vi "FTW-Test-Reflection-ConPaneInterface.vi"() -> (0 "Test Result":errorcluster)   [LabVIEW 2015]
uses:
  src/reflection/FTW-Reflection-Types.ctl
  src/reflection/core/FTW-Reflection-ConPaneInterface-Function.ctl
  src/reflection/core/FTW-Reflection-ConPaneInterface-Terminal.ctl
  src/reflection/FTW-Reflection-Type.vi
  src/error/FTW-ERR-Assert-DeveloperError.vi
  src/error/FTW-ERR-StatusOK.vi
  src/reflection/FTW-Reflection-TypeDescriptorToDefaultData.vi
  src/error/FTW-ERR-NoErrorConstant.vi
  src/error/FTW-ERR-ThrowInfo.vi
  src/error/FTW-ERR-ThrowError.vi
  src/reflection/FTW-Reflection-Array.vi
  src/error/FTW-ERR-CallChain.vi
  src/string/FTW-STR-ReplaceWhitespace.vi
  src/string/FTW-STR-Array-Delimit.vi
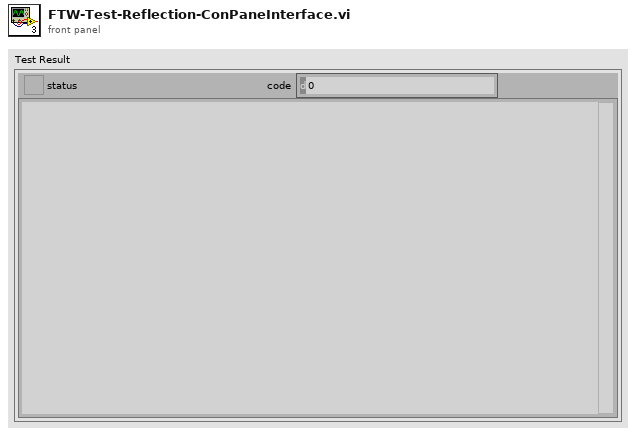
[diagram p1: front panel]
types:
  T1 = typedef "FTW-Reflection-ConPaneInterface-Terminal.ctl" = cluster{"Name":string, "LabVIEW Type":T2, "Datatype":variant, "Bounds":cluster{"Left":i32, "Top":i32, "Right":i32, "Bottom":i32}, "Input Stomp Index":i32, "Input":bool, "Wired":bool, "Dynamic Dispatch":bool, "Recommended":bool, "Required":bool, "Stomped":bool, "RSV20":bool, "RSV40":bool}
  T2 = typedef "FTW-Reflection-Types.ctl" = enum16{"Unknown", "Void", "Array", "Cluster", "LVObject", "Boolean", "I8", "I16", "I32", "I64", "U8", "U16", "U32", "U64", "SGL", "DBL", "EXT", "CSG", "CDB", "CXT", "FXP", "EnumU8", "EnumU16", "EnumU32", "EnumU64", "SGLwithUnit", "DBLwithUnit", "EXTwithUnit", "CSGwithUnit", "CDBwithUnit", "CXTwithUnit", "String", "Path", "Picture", "Tag", "LVVariant", "Timestamp", "WaveformI8", "WaveformI16", "WaveformI32", "WaveformI64", "WaveformU8", "WaveformU16", "WaveformU32", "WaveformU64", "WaveformSGL", "WaveformDBL", "WaveformEXT", "WaveformCSG", "WaveformCDB", "WaveformCXT", "WaveformDigital", "WaveformUnknownType", "DigitalData", "DynamicData", "ExternalData", "FileByteStream", "TDMStream", "dotNET", "ActiveX", "VIServerReference", "VIReference", "ApplicationInstance", "Menu", "ConnectionDataSocket", "ConnectionVISA", "ConnectionBluetooth", "ConnectionIrDA", "ConnectionTCP", "ConnectionUDP", "ConnectionHTTPClient", "ConnectionFTP", "Occurrence", "Notifier", "Queue", "Rendezvous", "Semaphore", "RTFIFO", "EventPublisher", "EventRegistration", "EventCallback", "DataValueReference", "GenericClass", "GenericClassTag", "GenericClassDeepCopy", "GenericClassFlattened", "GenericClassTagFlattened", "GenericReferenceType", "WindowsRegistry", "OverloadedDatalogRef", "ReferenceUnknownType", "ByteArray", "ConPaneInterface", "FTWObject"}
  T3 = typedef "FTW-Reflection-ConPaneInterface-Function.ctl" = cluster{"ConPane Code":i32, "ConPane Rotated":bool, "ConPane Flipped Horizontally":bool, "Asynchronous":bool, "Not a Pure Function (has side effects), or not SubRoutine":bool, "Subroutine Priority":bool, "Reserved 1":bool, "Reserved 2":bool, "Reserved 3":bool, "Reserved 4":bool, "Reserved 5":bool}
  T4 = cluster{i32, "ConPane Code":i32, "ConPane Rotated":bool, "ConPane Flipped Horizontally":bool}[]
  T5 = cluster{i32, "ConPane Code":i32, "ConPane Rotated":bool, "ConPane Flipped Horizontally":bool}
  T6 = cluster{"Name":string, "Wired":bool, "Required":bool, "Recommended":bool, "LabVIEW Type":T2}[]
  T7 = cluster{"Name":string, "Wired":bool, "Required":bool, "Recommended":bool, "LabVIEW Type":T2}
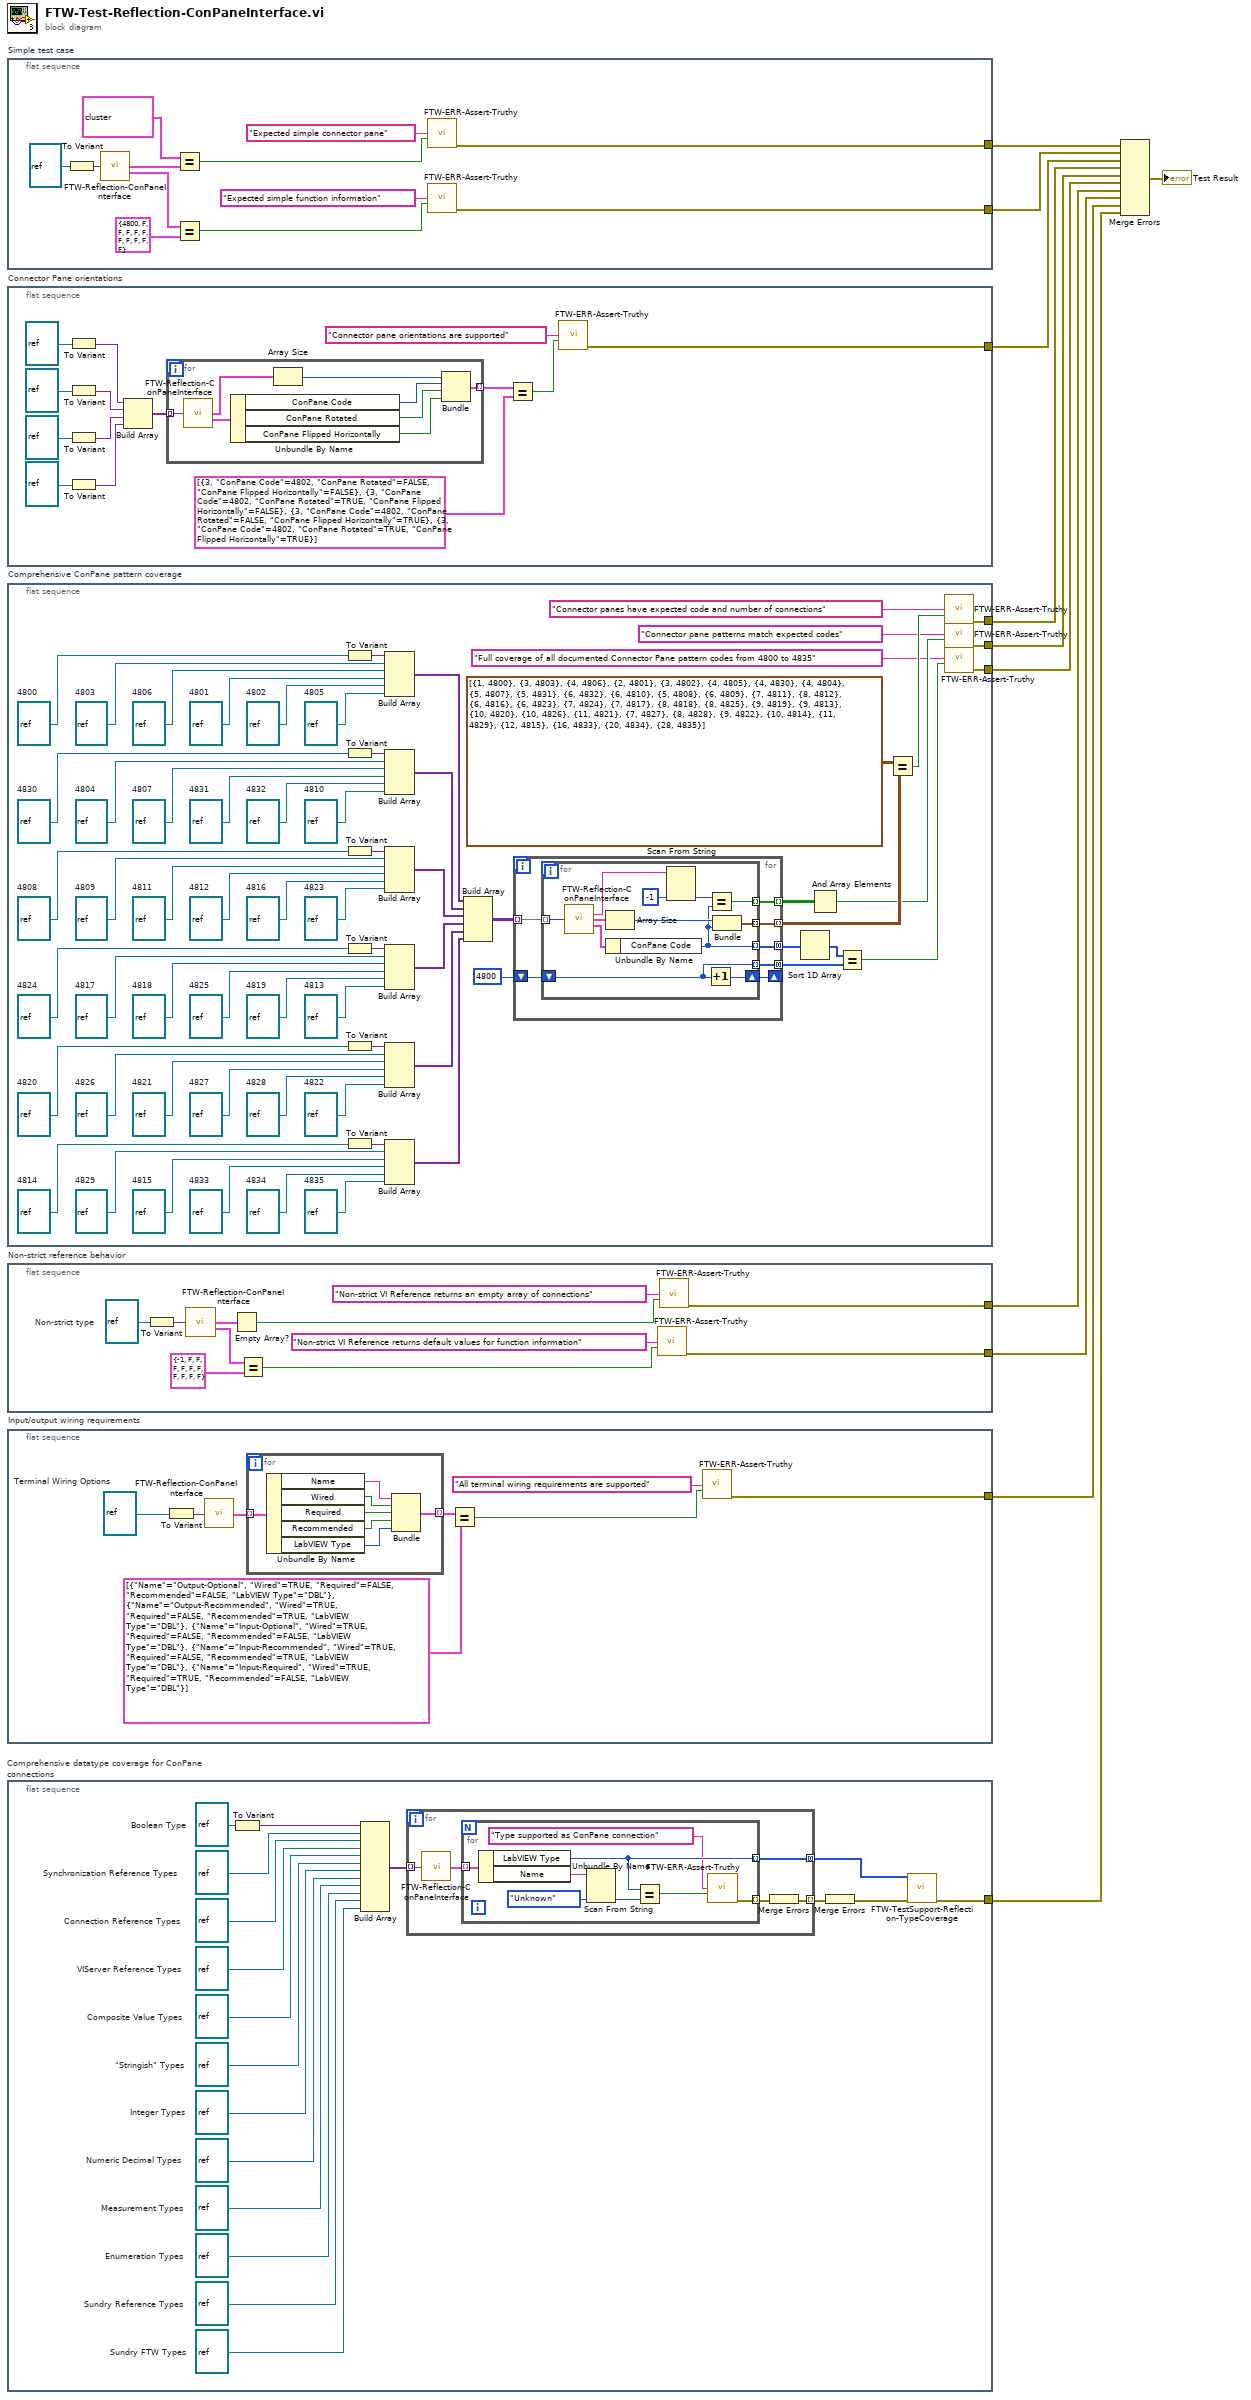
[diagram p0: block diagram]
diagram:
  n1 = flat-sequence "Simple test case" {
    tunnel: [w15] -> w11
    tunnel: [w12] -> w10
    frame #0 {
      n2 = To Variant(anything=refnum<vi> refnum) -> (Variant=w18:variant)
      n3 = call "FTW-Reflection-ConPaneInterface.vi"("VI Connector Pane (or VI Reference)"=w18) -> ("Terminals"=w23:T1[], "Function Information"=w21:T3)  [unwired: 12 in, 1 out]
      n4 = Equal?(x=T1[] [{"Name"="", "LabVIEW Type"=enum."Unknown", "Datatype"=variant, "Bounds"={"Left"=0, "Top"=0, "Right"=32, "Bottom"=32}, "Input Stomp Index"=-1, "Input"=FALSE, "Wired"=FALSE, "Dynamic Dispatch"=FALSE, "Recommended"=FALSE, "Required"=FALSE, "Stomped"=FALSE, "RSV20"=FALSE, "RSV40"=FALSE}] ("Terminals"), y=w23) -> (x = y?=w17:bool)
      n5 = Equal?(x=w21, y=T3 {"ConPane Code"=4800, "ConPane Rotated"=FALSE, "ConPane Flipped Horizontally"=FALSE, "Asynchronous"=FALSE, "Not a Pure Function (has side effects), or not SubRoutine"=FALSE, "Subroutine Priority"=FALSE, "Reserved 1"=FALSE, "Reserved 2"=FALSE, "Reserved 3"=FALSE, "Reserved 4"=FALSE, "Reserved 5"=FALSE} ("Function Information")) -> (x = y?=w13:bool)
      n6 = call "FTW-ERR-Assert-Truthy.vi"("Assertion"="Expected simple connector pane", "Assertion holds true?"=w17) -> ("error out"=w15:errorcluster)  [unwired: 13 in]
      n7 = call "FTW-ERR-Assert-Truthy.vi"("Assertion"="Expected simple function information", "Assertion holds true?"=w13) -> ("error out"=w12:errorcluster)  [unwired: 13 in]
    }
  }
  n8 = flat-sequence "Connector Pane orientations" {
    tunnel: [w24] -> w9
    frame #0 {
      n9 = To Variant(anything=refnum<vi> refnum) -> (Variant=w35:variant)
      n10 = To Variant(anything=refnum<vi> refnum) -> (Variant=w31:variant)
      n11 = To Variant(anything=refnum<vi> refnum) -> (Variant=w30:variant)
      n12 = To Variant(anything=refnum<vi> refnum) -> (Variant=w29:variant)
      n13 = Build Array(w35, w31, w30, w29) -> (w36:variant[])
      n14 = for {
        tunnel: [w41] -> w28 mode=indexing
        tunnel: w36 -> [w40] mode=indexing
        n15 = call "FTW-Reflection-ConPaneInterface.vi"("VI Connector Pane (or VI Reference)"=w40) -> ("Terminals"=w38:T1[], "Function Information"=w39:T3)  [unwired: 12 in, 1 out]
        n16 = Unbundle By Name(w39) -> ("ConPane Code"=w44:i32, "ConPane Rotated"=w43:bool, "ConPane Flipped Horizontally"=w42:bool)
        n17 = Array Size(array=w38) -> (size(s)=w45:i32)
        n18 = Bundle(w45, "ConPane Code"=w44, "ConPane Rotated"=w43, "ConPane Flipped Horizontally"=w42) -> (w41:T5)  [unwired: 1 in]
      }
      n19 = Equal?(x=w28, y=T4 [{3, "ConPane Code"=4802, "ConPane Rotated"=FALSE, "ConPane Flipped Horizontally"=FALSE}, {3, "ConPane Code"=4802, "ConPane Rotated"=TRUE, "ConPane Flipped Horizontally"=FALSE}, {3, "ConPane Code"=4802, "ConPane Rotated"=FALSE, "ConPane Flipped Horizontally"=TRUE}, {3, "ConPane Code"=4802, "ConPane Rotated"=TRUE, "ConPane Flipped Horizontally"=TRUE}] ("Array")) -> (x = y?=w25:bool)
      n20 = call "FTW-ERR-Assert-Truthy.vi"("Assertion"="Connector pane orientations are supported", "Assertion holds true?"=w25) -> ("error out"=w24:errorcluster)  [unwired: 13 in]
    }
  }
  n21 = flat-sequence "Comprehensive ConPane pattern coverage" {
    tunnel: [w48] -> w8
    tunnel: [w47] -> w7
    tunnel: [w46] -> w6
    frame #0 {
      w81 = refnum<vi> refnum  # 4835
      w86 = refnum<vi> refnum  # 4822
      w82 = refnum<vi> refnum  # 4834
      w87 = refnum<vi> refnum  # 4828
      w83 = refnum<vi> refnum  # 4833
      w88 = refnum<vi> refnum  # 4827
      w84 = refnum<vi> refnum  # 4815
      w89 = refnum<vi> refnum  # 4821
      w85 = refnum<vi> refnum  # 4829
      w90 = refnum<vi> refnum  # 4826
      w74 = refnum<vi> refnum  # 4814
      w73 = refnum<vi> refnum  # 4820
      w91 = refnum<vi> refnum  # 4813
      w96 = refnum<vi> refnum  # 4823
      w92 = refnum<vi> refnum  # 4819
      w97 = refnum<vi> refnum  # 4816
      w93 = refnum<vi> refnum  # 4825
      w98 = refnum<vi> refnum  # 4812
      w94 = refnum<vi> refnum  # 4818
      w99 = refnum<vi> refnum  # 4811
      w95 = refnum<vi> refnum  # 4817
      w100 = refnum<vi> refnum  # 4809
      w72 = refnum<vi> refnum  # 4824
      w71 = refnum<vi> refnum  # 4808
      w101 = refnum<vi> refnum  # 4810
      w106 = refnum<vi> refnum  # 4805
      w102 = refnum<vi> refnum  # 4832
      w107 = refnum<vi> refnum  # 4802
      w103 = refnum<vi> refnum  # 4831
      w108 = refnum<vi> refnum  # 4801
      w104 = refnum<vi> refnum  # 4807
      w109 = refnum<vi> refnum  # 4806
      w105 = refnum<vi> refnum  # 4804
      w110 = refnum<vi> refnum  # 4803
      w70 = refnum<vi> refnum  # 4830
      w62 = refnum<vi> refnum  # 4800
      n22 = To Variant(anything=w62) -> (Variant=w63:variant)
      n23 = To Variant(anything=w70) -> (Variant=w69:variant)
      n24 = To Variant(anything=w71) -> (Variant=w68:variant)
      n25 = To Variant(anything=w72) -> (Variant=w67:variant)
      n26 = To Variant(anything=w73) -> (Variant=w66:variant)
      n27 = To Variant(anything=w74) -> (Variant=w65:variant)
      n28 = Build Array(w63, w110, w109, w108, w107, w106) -> (w80:variant[])
      n29 = Build Array(w69, w105, w104, w103, w102, w101) -> (w79:variant[])
      n30 = Build Array(w68, w100, w99, w98, w97, w96) -> (w78:variant[])
      n31 = Build Array(w67, w95, w94, w93, w92, w91) -> (w77:variant[])
      n32 = Build Array(w66, w90, w89, w88, w87, w86) -> (w76:variant[])
      n33 = Build Array(w65, w85, w84, w83, w82, w81) -> (w75:variant[])
      n34 = Build Array(w80, w79, w78, w77, w76, w75) -> (w64:variant[][])
      n35 = for {
        tunnel: w64 -> [w117] mode=indexing
        tunnel: [w116] -> w56 mode=indexing
        tunnel: [w115] -> w61 mode=concatenating
        shift-right: [w113] -> _
        shift-left: 4800 ("ConPane Code") -> [w114]
        tunnel: [w112] -> w58 mode=concatenating
        tunnel: [w111] -> w55 mode=indexing
        n36 = for {
          tunnel: w117 -> [w129] mode=indexing
          tunnel: [w125] -> w116 mode=indexing
          tunnel: [w119] -> w115 mode=indexing
          shift-right: [w124] -> w113
          shift-left: w114 -> [w123]
          tunnel: [w123] -> w112 mode=indexing
          tunnel: [w118] -> w111 mode=indexing
          n37 = call "FTW-Reflection-ConPaneInterface.vi"("VI Connector Pane (or VI Reference)"=w129) -> ("Data Name"=w122:string, "Terminals"=w128:T1[], "Function Information"=w127:T3)  [unwired: 12 in]
          n38 = Array Size(array=w128) -> (size(s)=w126:i32)
          n39 = Unbundle By Name(w127) -> ("ConPane Code"=w119:i32)
          n40 = Scan From String(input string=w122, default 1=-1 ("default value 1")) -> (output 1=w120:i32)  [unwired: 3 in, 3 out]
          n41 = Increment(x=w123) -> (x+1=w124:i32)
          n42 = Equal?(x=w120, y=w119) -> (x = y?=w118:bool)
          n43 = Bundle(w126, "ConPane Code"=w119) -> (w125:cluster{i32, "ConPane Code":i32})  [unwired: 1 in]
        }
      }
      n44 = Sort 1D Array(array=w61) -> (sorted array=w59:i32[])
      n45 = And Array Elements(Boolean array=w55) -> (logical AND=w52:bool)
      n46 = Equal?(x=w59, y=w58) -> (x = y?=w50:bool)
      n47 = Equal?(x=cluster{i32, i32}[][] [[{1, 4800}, {3, 4803}, {4, 4806}, {2, 4801}, {3, 4802}, {4, 4805}], [{4, 4830}, {4, 4804}, {5, 4807}, {5, 4831}, {6, 4832}, {6, 4810}], [{5, 4808}, {6, 4809}, {7, 4811}, {8, 4812}, {6, 4816}, {6, 4823}], [{7, 4824}, {7, 4817}, {8, 4818}, {8, 4825}, {9, 4819}, {9, 4813}], [{10, 4820}, {10, 4826}, {11, 4821}, {7, 4827}, {8, 4828}, {9, 4822}], [{10, 4814}, {11, 4829}, {12, 4815}, {16, 4833}, {20, 4834}, {28, 4835}]], y=w56) -> (x = y?=w53:bool)
      n48 = call "FTW-ERR-Assert-Truthy.vi"("Assertion"="Connector panes have expected code and number of connections", "Assertion holds true?"=w53) -> ("error out"=w48:errorcluster)  [unwired: 13 in]
      n49 = call "FTW-ERR-Assert-Truthy.vi"("Assertion"="Connector pane patterns match expected codes", "Assertion holds true?"=w52) -> ("error out"=w47:errorcluster)  [unwired: 13 in]
      n50 = call "FTW-ERR-Assert-Truthy.vi"("Assertion"="Full coverage of all documented Connector Pane pattern codes from 4800 to 4835", "Assertion holds true?"=w50) -> ("error out"=w46:errorcluster)  [unwired: 13 in]
    }
  }
  n51 = flat-sequence "Non-strict reference behavior" {
    tunnel: [w131] -> w5
    tunnel: [w130] -> w4
    frame #0 {
      w140 = refnum<vi> refnum  # Non-strict type
      n52 = To Variant(anything=w140) -> (Variant=w139:variant)
      n53 = call "FTW-Reflection-ConPaneInterface.vi"("VI Connector Pane (or VI Reference)"=w139) -> ("Terminals"=w138:T1[], "Function Information"=w136:T3)  [unwired: 12 in, 1 out]
      n54 = Empty Array?(array=w138) -> (empty?=w135:bool)
      n55 = Equal?(x=w136, y=T3 {"ConPane Code"=-1, "ConPane Rotated"=FALSE, "ConPane Flipped Horizontally"=FALSE, "Asynchronous"=FALSE, "Not a Pure Function (has side effects), or not SubRoutine"=FALSE, "Subroutine Priority"=FALSE, "Reserved 1"=FALSE, "Reserved 2"=FALSE, "Reserved 3"=FALSE, "Reserved 4"=FALSE, "Reserved 5"=FALSE} ("Function Information")) -> (x = y?=w133:bool)
      n56 = call "FTW-ERR-Assert-Truthy.vi"("Assertion"="Non-strict VI Reference returns default values for function information", "Assertion holds true?"=w133) -> ("error out"=w130:errorcluster)  [unwired: 13 in]
      n57 = call "FTW-ERR-Assert-Truthy.vi"("Assertion"="Non-strict VI Reference returns an empty array of connections", "Assertion holds true?"=w135) -> ("error out"=w131:errorcluster)  [unwired: 13 in]
    }
  }
  n58 = flat-sequence "Input/output wiring requirements" {
    tunnel: [w141] -> w3
    frame #0 {
      w147 = refnum<vi> refnum  # Terminal Wiring Options
      n59 = To Variant(anything=w147) -> (Variant=w146:variant)
      n60 = call "FTW-Reflection-ConPaneInterface.vi"("VI Connector Pane (or VI Reference)"=w146) -> ("Terminals"=w148:T1[])  [unwired: 12 in, 2 out]
      n61 = for {
        tunnel: w148 -> [w155] mode=indexing
        tunnel: [w150] -> w145 mode=indexing
        n62 = Unbundle By Name(w155) -> ("Name"=w154:string, "Wired"=w149:bool, "Required"=w153:bool, "Recommended"=w152:bool, "LabVIEW Type"=w151:T2)
        n63 = Bundle("Name"=w154, "Wired"=w149, "Required"=w153, "Recommended"=w152, "LabVIEW Type"=w151) -> (w150:T7)  [unwired: 1 in]
      }
      n64 = Equal?(x=w145, y=T6 [{"Name"="Output-Optional", "Wired"=TRUE, "Required"=FALSE, "Recommended"=FALSE, "LabVIEW Type"=enum."DBL"}, {"Name"="Output-Recommended", "Wired"=TRUE, "Required"=FALSE, "Recommended"=TRUE, "LabVIEW Type"=enum."DBL"}, {"Name"="Input-Optional", "Wired"=TRUE, "Required"=FALSE, "Recommended"=FALSE, "LabVIEW Type"=enum."DBL"}, {"Name"="Input-Recommended", "Wired"=TRUE, "Required"=FALSE, "Recommended"=TRUE, "LabVIEW Type"=enum."DBL"}, {"Name"="Input-Required", "Wired"=TRUE, "Required"=TRUE, "Recommended"=FALSE, "LabVIEW Type"=enum."DBL"}] ("Array")) -> (x = y?=w143:bool)
      n65 = call "FTW-ERR-Assert-Truthy.vi"("Assertion"="All terminal wiring requirements are supported", "Assertion holds true?"=w143) -> ("error out"=w141:errorcluster)  [unwired: 13 in]
    }
  }
  n66 = flat-sequence "Comprehensive datatype coverage for ConPane connections" {
    tunnel: [w160] -> w2
    frame #0 {
      w156 = refnum<vi> refnum  # Sundry FTW Types
      w161 = refnum<vi> refnum  # Sundry Reference Types
      w162 = refnum<vi> refnum  # Enumeration Types
      w164 = refnum<vi> refnum  # Boolean Type
      w166 = refnum<vi> refnum  # Measurement Types
      w167 = refnum<vi> refnum  # Numeric Decimal Types
      w168 = refnum<vi> refnum  # Integer Types
      w169 = refnum<vi> refnum  # "Stringish" Types
      w170 = refnum<vi> refnum  # Composite Value Types
      w171 = refnum<vi> refnum  # VIServer Reference Types
      w172 = refnum<vi> refnum  # Connection Reference Types
      w165 = refnum<vi> refnum  # Synchronization Reference Types
      n67 = To Variant(anything=w164) -> (Variant=w163:variant)
      n68 = Build Array(w163, w165, w172, w171, w170, w169, w168, w167, w166, w162, w161, w156) -> (w173:variant[])
      n69 = for {
        tunnel: [w176] -> w159 mode=concatenating
        tunnel: w173 -> [w178] mode=indexing
        tunnel: [w174] -> w158 mode=indexing
        n70 = call "FTW-Reflection-ConPaneInterface.vi"("VI Connector Pane (or VI Reference)"=w178) -> ("Terminals"=w177:T1[])  [unwired: 12 in, 2 out]
        n71 = for {
          tunnel: w177 -> [w186] mode=indexing
          tunnel: [w182] -> w176 mode=indexing
          tunnel: [w179] -> w175 mode=indexing
          n72 = Unbundle By Name(w186) -> ("LabVIEW Type"=w182:T2, "Name"=w183:string)
          n73 = Scan From String(input string=w183, default 1=FTW-Reflection-Types."Unknown" ("Element Type")) -> (output 1=w184:T2)  [unwired: 3 in, 3 out]
          n74 = Equal?(x=w182, y=w184) -> (x = y?=w181:bool)
          n75 = call "FTW-ERR-Assert-Truthy.vi"("Assertion"="Type supported as ConPane connection", "Assertion holds true?"=w181) -> ("error out"=w179:errorcluster)  [unwired: 13 in]
        }
        n76 = Merge Errors(w175) -> (w174:errorcluster)
      }
      n77 = Merge Errors(w158) -> (w157:errorcluster)
      n78 = call "FTW-TestSupport-Reflection-TypeCoverage.vi"("Types Tested"=w159, "error in"=w157) -> ("error out"=w160:errorcluster)  [unwired: 13 in]
    }
  }
  n79 = Merge Errors(w11, w10, w9, w8, w7, w6, w5, w4, w3, w2) -> (→"Test Result":errorcluster)
